vi "RefClass_Probe.vi"(1 "LabVIEW Object":refnum<class>) -> (0 "Boolean":bool)   [LabVIEW 2016]
panel:
  out "Text":cluster{"Text":string}
  out "error out":errorcluster
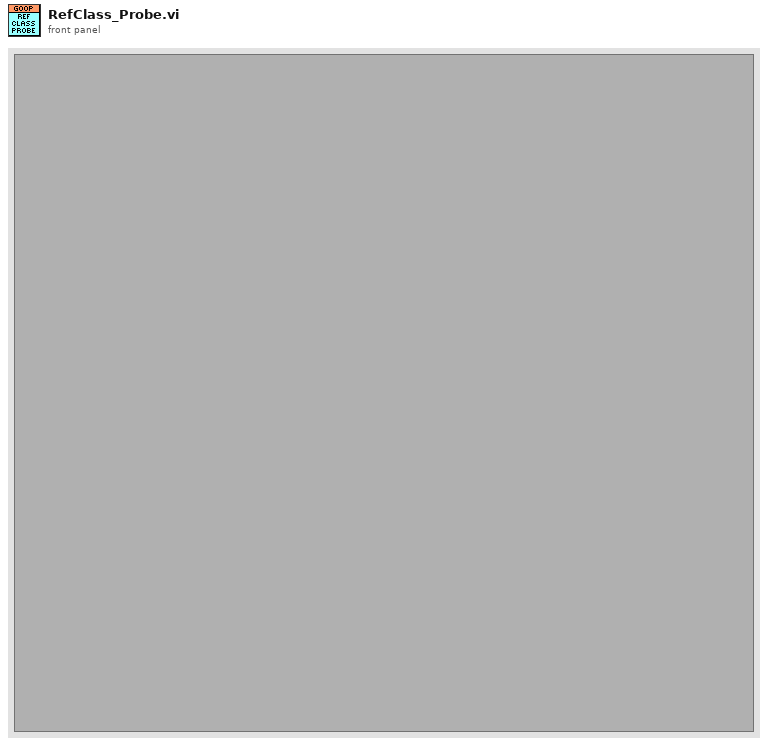
[diagram p1: front panel]
types:
  T1 = cluster{"ClassNames":string[], "ObjectAttributes":path[], "MD5":string, "CacheVI-Name":string, "Refs":u32[], "CacheVI":path}
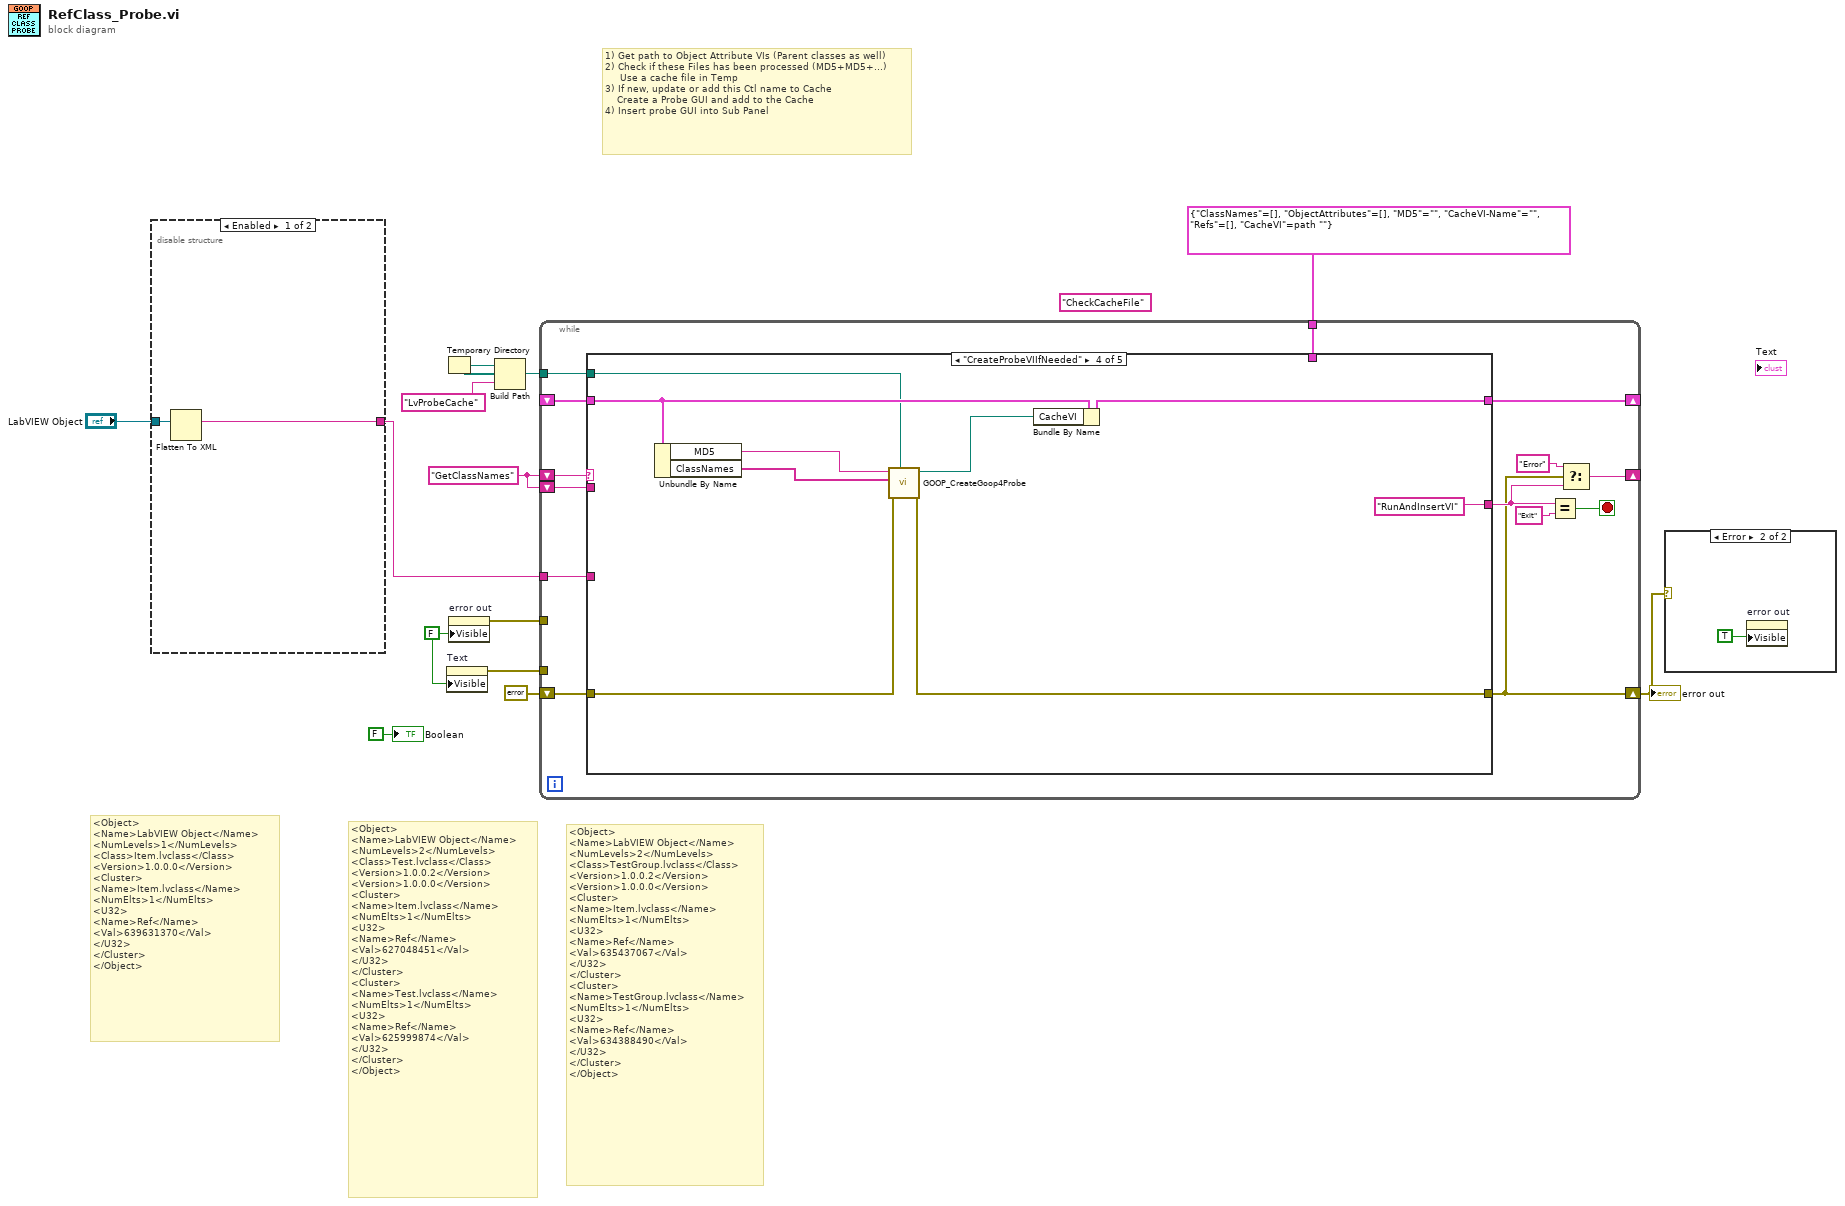
[diagram p0: block diagram]
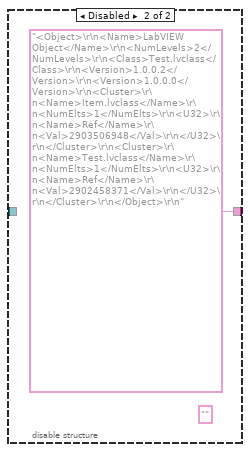
[diagram p3: hidden frame]
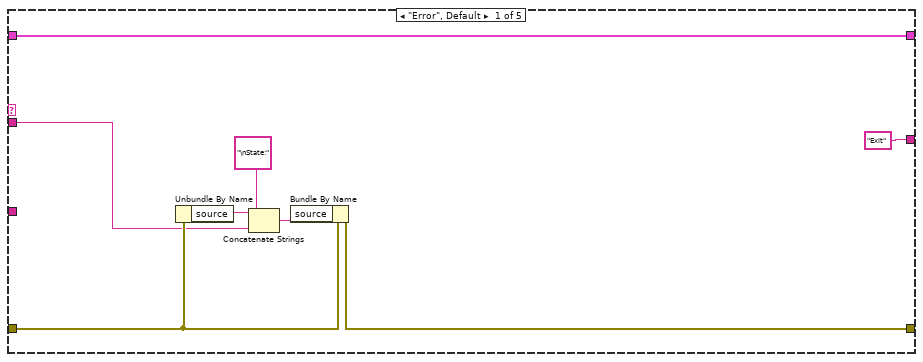
[diagram p4: hidden frame]
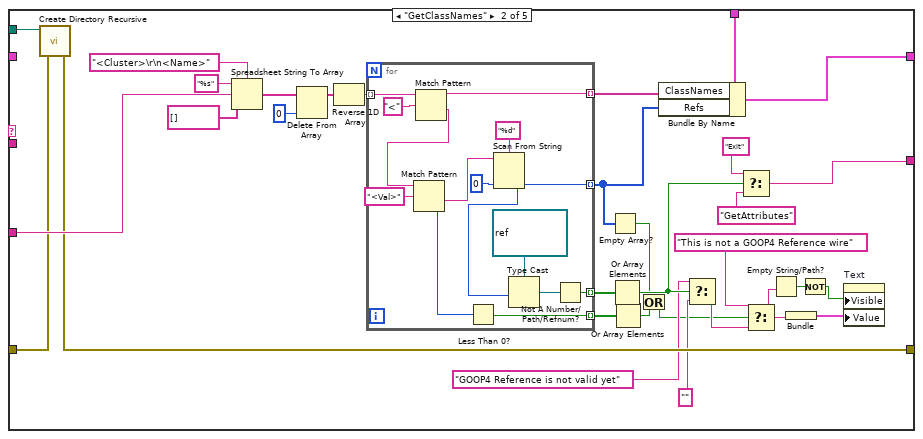
[diagram p5: hidden frame]
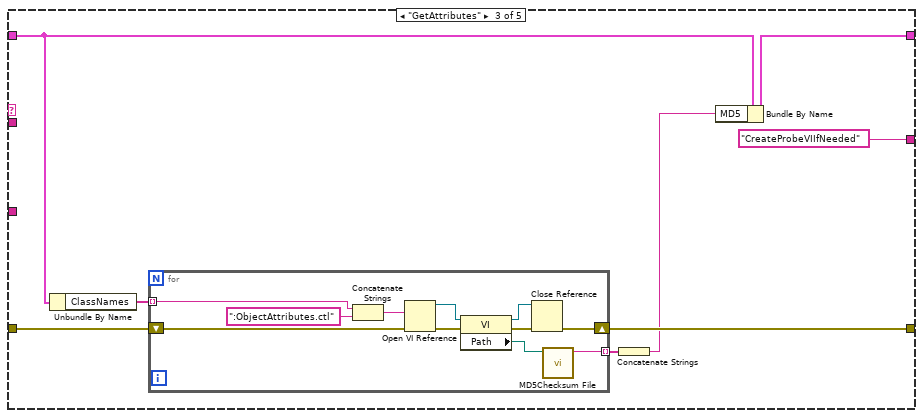
[diagram p6: hidden frame]
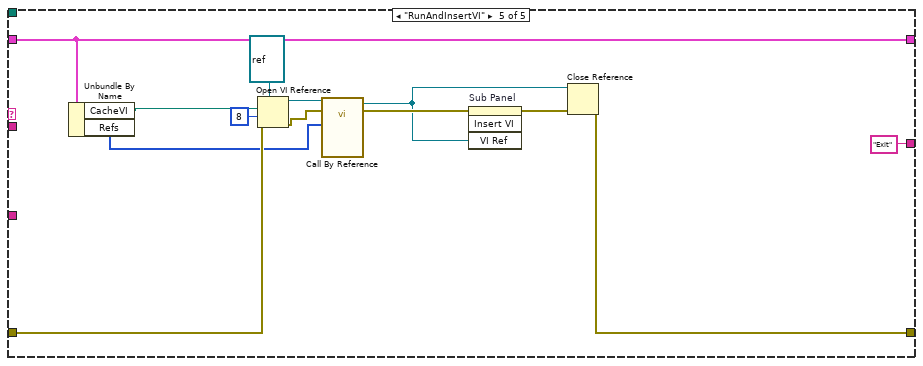
[diagram p7: hidden frame]
diagram:
  (unwired) "CheckCacheFile"
  w2 = FALSE ("Visible")
  w3 = "GetClassNames"
  # "<Object>\n<Name>LabVIEW Object</Name>\n<NumLevels>1</NumLevels>\n<Class>Item.lvclass</Class>\n<Version>1.0.0.0</Version>\n<Cluster>\n<Name>Item.lvclass</Name>\n<NumElts>1</NumElts>\n<U32>\n<Name>Ref</Name>\n<Val>639631370</Val>\n</U32>\n</Cluster>\n</Object>"
  # "<Object>\n<Name>LabVIEW Object</Name>\n<NumLevels>2</NumLevels>\n<Class>TestGroup.lvclass</Class>\n<Version>1.0.0.2</Version>\n<Version>1.0.0.0</Version>\n<Cluster>\n<Name>Item.lvclass</Name>\n<NumElts>1</NumElts>\n<U32>\n<Name>Ref</Name>\n<Val>635437067</Val>\n</U32>\n</Cluster>\n<Cluster>\n<Name>TestGroup.lvclass</Name>\n<NumElts>1</NumElts>\n<U32>\n<Name>Ref</Name>\n<Val>634388490</Val>\n</U32>\n</Cluster>\n</Object>"
  # "<Object>\n<Name>LabVIEW Object</Name>\n<NumLevels>2</NumLevels>\n<Class>Test.lvclass</Class>\n<Version>1.0.0.2</Version>\n<Version>1.0.0.0</Version>\n<Cluster>\n<Name>Item.lvclass</Name>\n<NumElts>1</NumElts>\n<U32>\n<Name>Ref</Name>\n<Val>627048451</Val>\n</U32>\n</Cluster>\n<Cluster>\n<Name>Test.lvclass</Name>\n<NumElts>1</NumElts>\n<U32>\n<Name>Ref</Name>\n<Val>625999874</Val>\n</U32>\n</Cluster>\n</Object>"
  # "1) Get path to Object Attribute VIs (Parent classes as well)\n2) Check if these Files has been processed (MD5+MD5+...)\n     Use a cache file in Temp\n3) If new, update or add this Ctl name to Cache\n    Create a Probe GUI and add to the Cache\n4) Insert probe GUI into Sub Panel"
  n1 = disable-structure shown="Enabled" {
    disable-tunnel: [w15 "<Object>\r\n<Name>LabVIEW Object</Name>\r\n<NumLevels>2</NumLevels>\r\n<Class>Test.lvclass</Class>\r\n<Version>1.0.0.2</Version>\r\n<Version>1.0.0.0</Version>\r\n<Cluster>\r\n<Name>Item.lvclass</Name>\r\n<NumElts>1</NumElts>\r\n<U32>\r\n<Name>Ref</Name>\r\n<Val>2903506948</Val>\r\n</U32>\r\n</Cluster>\r\n<Cluster>\r\n<Name>Test.lvclass</Name>\r\n<NumElts>1</NumElts>\r\n<U32>\r\n<Name>Ref</Name>\r\n<Val>2902458371</Val>\r\n</U32>\r\n</Cluster>\r\n</Object>\r\n" ("String")] -> w12
    disable-tunnel: "LabVIEW Object" -> [w14 _]
    frame Enabled {
      n2 = Flatten To XML(anything=w14) -> (xml string=w15:string)
    }
    frame Disabled {
      (unwired) "" ("String")
    }
  }
  n3 = Temporary Directory() -> (w9:path)
  n4 = property on="Text" class="Clust (strict)"("Visible"=w2) -> (error out=w1:errorcluster)  [unwired: 2 in, 1 out]
  n5 = property on="error out" class="Clust (strict)"("Visible"=w2) -> (error out=w5:errorcluster)  [unwired: 2 in, 1 out]
  n6 = Build Path(base path=w9, name or relative path="LvProbeCache") -> (appended path=w7:path)
  n7 = while {
    shift-right: [w23] -> w4
    shift-left: errorcluster {"status"=FALSE, "code"=0, "source"=""} ("error IO") -> [w30]
    shift-right: [w28] -> _
    shift-left: w3 -> [w29]
    shift-right: [w22] -> _
    shift-left: _ -> [w21]
    tunnel: T1 {"ClassNames"=[], "ObjectAttributes"=[], "MD5"="", "CacheVI-Name"="", "Refs"=[], "CacheVI"=path ""} -> [w20]
    tunnel: w12 -> [w19]
    tunnel: w7 -> [w18]
    tunnel: w5 -> [_]
    shift-left: w3 -> [w17]
    tunnel: w1 -> [_]
    stop <- w27 stop-if-true
    n8 = case shown="\"CreateProbeVIIfNeeded\"" w29 {
      tunnel: w30 -> [w36 w60 w90 w112 w125]
      tunnel: [w35 w59 w89 w111 w116] -> w23
      tunnel: ["Exit" w56 "CreateProbeVIIfNeeded" "RunAndInsertVI" "Exit"] -> w24
      tunnel: [w37 w70 w88 w105 w119] -> w22
      tunnel: w21 -> [w37 _ w92 w110 w119]
      tunnel: w20 -> [_ w69 _ _ _]
      tunnel: w19 -> [_ w66 _ _ _]
      tunnel: w18 -> [_ w61 _ w106 _]
      tunnel: w17 -> [w32 _ _ _ _]
      frame "Error", Default {
        n9 = Unbundle By Name(w36) -> ("source"=w34:string)
        n10 = Concatenate Strings(w34, "\nState:" ("string"), w32) -> (w33:string)
        n11 = Bundle By Name(cluster=w36, "source"=w33) -> (w35:errorcluster)
      }
      frame "GetClassNames" {
        n12 = call <vilib>:"Create Directory Recursive.vi"("error in (no error)"=w60, "directory"=w61) -> ("error out"=w59:errorcluster)  [unwired: 3 in, 2 out]
        n13 = Spreadsheet String To Array(delimiter (Tab)="<Cluster>\r\n<Name>", format string="%s", spreadsheet string=w66, array type (2D Dbl)=string[] []) -> (array=w65:string[])
        n14 = Delete From Array(array=w65, index=0) -> (array with subset deleted=w62:string[])  [unwired: 1 in, 1 out]
        n15 = Reverse 1D Array(array=w62) -> (reversed array=w53:string[])
        n16 = for {
          tunnel: w53 -> [w84] mode=indexing
          tunnel: [w82] -> w54 mode=indexing
          tunnel: [w74] -> w42 mode=indexing
          tunnel: [w73] -> w55 mode=indexing
          tunnel: [w71] -> w52 mode=indexing
          n17 = Match Pattern(string=w84, regular expression="<") -> (before substring=w82:string, after substring=w77:string)  [unwired: 1 in, 2 out]
          n18 = Match Pattern(string=w77, regular expression="<Val>") -> (after substring=w78:string, offset past match=w72:i32)  [unwired: 1 in, 2 out]
          n19 = Less Than 0?(x=w72) -> (x < 0?=w71:bool)
          n20 = Scan From String(format string="%d", input string=w78, default 1=u32 0 ("default value 1")) -> (output 1=w74:u32)  [unwired: 2 in, 3 out]
          n21 = Type Cast(type=refnum<data-value> refnum ("data value reference"), x=w74) -> (*(type *) &x=w75:refnum<data-value>)
          n22 = Not A Number/Path/Refnum?(number/path/refnum=w75) -> (NaN/Path/Refnum?=w73:bool)
        }
        n23 = Empty Array?(array=w42) -> (empty?=w39:bool)
        n24 = Or Array Elements(Boolean array=w55) -> (logical OR=w48:bool)
        n25 = Or Array Elements(Boolean array=w52) -> (logical OR=w41:bool)
        n26 = Or(x=w39, y=w41) -> (x .or. y?=w40:bool)
        n27 = Bundle By Name(cluster=w69, "ClassNames"=w54, "Refs"=w42) -> (w70:T1)
        n28 = Select(t="GOOP4 Reference is not valid yet", s=w48, f="") -> (s? t:f=w49:string)
        n29 = Select(t="Exit", s=w48, f="GetAttributes") -> (s? t:f=w56:string)
        n30 = Select(t="This is not a GOOP4 Reference wire", s=w40, f=w49) -> (s? t:f=w45:string)
        n31 = Empty String/Path?(string/path=w45) -> (empty?=w44:bool)
        n32 = Bundle(w45) -> (w51:cluster{string})  [unwired: 1 in]
        n33 = Not(x=w44) -> (.not. x?=w43:bool)
        n34 = property on="Text" class="Clust (strict)"("Visible"=w43, "Value"=w51) -> ()  [unwired: 2 in, 2 out]
      }
      frame "GetAttributes" {
        n35 = Unbundle By Name(w92) -> ("ClassNames"=w91:string[])
        n36 = for {
          tunnel: w91 -> [w95] mode=indexing
          shift-right: [w97] -> w89
          shift-left: w90 -> [w96]
          tunnel: [w93] -> w87 mode=indexing
          n37 = Concatenate Strings(w95, ":ObjectAttributes.ctl" ("string")) -> (w102:string)
          n38 = Open VI Reference(vi path=w102, error in (no error)=w96) -> (vi reference=w101:refnum<vi>, error out=w100:errorcluster)  [unwired: 4 in]
          n39 = property class="VI"(reference=w101, error in=w100) -> (reference out=w98:refnum<vi>, error out=w99:errorcluster, "Path"=w94:path)
          n40 = Close Reference(reference=w98, error in (no error)=w99) -> (error out=w97:errorcluster)
          n41 = call <vilib>:"MD5Checksum File.vi"("Path"=w94) -> ("MD5 message-digest"=w93:string)  [unwired: 9 in, 1 out]
        }
        n42 = Concatenate Strings(w87) -> (w86:string)
        n43 = Bundle By Name(cluster=w92, "MD5"=w86) -> (w88:T1)
      }
      frame "CreateProbeVIIfNeeded" {
        n44 = Unbundle By Name(w110) -> ("MD5"=w107:string, "ClassNames"=w108:string[])
        n45 = call <userlib>:"GOOP_CreateGoop4Probe.vi"("LVProbeTemp"=w106, "error in (no error)"=w112, "ClassNames"=w108, "MD5"=w107) -> ("error out"=w111:errorcluster, "CacheVI-NameOut"=w104:path)  [unwired: 6 in]
        n46 = Bundle By Name(cluster=w110, "CacheVI"=w104) -> (w105:T1)
      }
      frame "RunAndInsertVI" {
        n47 = Unbundle By Name(w119) -> ("CacheVI"=w113:path, "Refs"=w114:u32[])
        n48 = Open VI Reference(type specifier VI Refnum (for type only)=refnum<vi> refnum, vi path=w113, options=8, error in (no error)=w125) -> (vi reference=w123:refnum<vi>, error out=w122:errorcluster)  [unwired: 2 in]
        n49 = call-by-ref "?"(reference=w123, error in=w122, "Refs"=w114) -> (reference out=w115:refnum<vi>, error out=w120:errorcluster)  [unwired: 11 in]
        n50 = invoke on="Sub Panel" class="SubPanel" method="Insert VI"(error in=w120, "VI Ref"=w115) -> (error out=w117:errorcluster)  [unwired: 2 in, 3 out]
        n51 = Close Reference(reference=w115, error in (no error)=w117) -> (error out=w116:errorcluster)
      }
    }
    n52 = Equal?(x=w24, y="Exit") -> (x = y?=w27:bool)
    n53 = Select(t="Error", s=w23, f=w24) -> (s? t:f=w28:string)
  }
  "error out" <- w4
  n54 = case shown="Error" w4 {
    frame No Error {
    }
    frame Error {
      n55 = property on="error out" class="Clust (strict)"("Visible"=TRUE) -> ()  [unwired: 2 in, 2 out]
    }
  }
  "Boolean" <- FALSE ("Boolean")
